vi "queryRV.vi"(0 "连接ID":refnum<k5>) -> (1 "连接ID输出":refnum<k5>, 2 "rv":dbl)   [LabVIEW 2017]
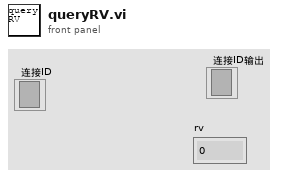
[diagram p1: front panel]
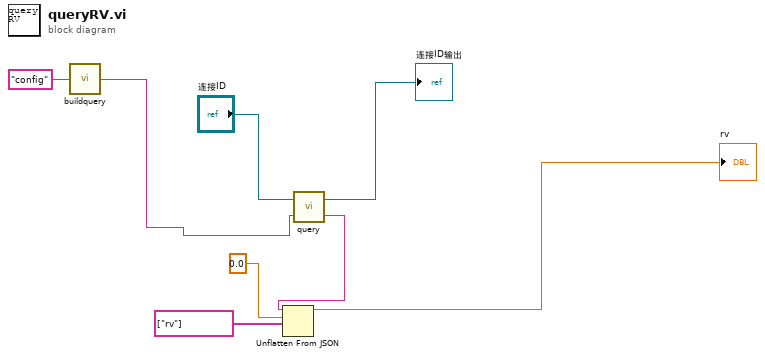
[diagram p0: block diagram]
diagram:
  n1 = call "buildquery.vi"("String"="config") -> ("JSON字符串"=w4:string)
  n2 = call "query.vi"("数据输入"=w4, "连接ID"="连接ID") -> ("数据输出"=w3:string, "连接ID输出"=→"连接ID输出":refnum<k5>)
  n3 = Unflatten From JSON(path=string[] ["rv"] ("路径"), JSON string=w3, type and defaults=0.0 ("rv 2")) -> (value=→"rv":dbl)  [unwired: 4 in, 1 out]
